vi "Reorder Analyzers Dialog.vi"(8 "error in":errorcluster, 11 "Analyzers.Process Cache":refnum<class "Controller Array.lvclass">) -> (0 "error out":errorcluster, 3 "Reordered Analyzers.Process Cache":refnum<class "Controller Array.lvclass">)   [LabVIEW 2020, in "RxnRover.lvlib"]
uses:
  RxnRover.lvlib
  Plugin Servers/Controller Array/Controller Array.lvclass
  Plugin Servers/Controller/Generic Plugin.lvclass/Generic Plugin.ctl
  Plugin Servers/Controller Array/Searchable Properties.ctl
  Plugin Servers/Controller/Generic Plugin.lvclass
panel:
  in  "Analyzer List":i32(listbox)
  out "Current Analyzer":string
  in  "Done":bool
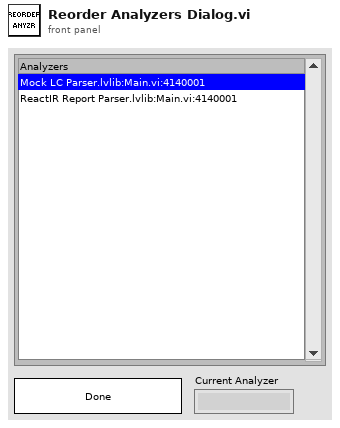
[diagram p1: front panel]
types:
  T1 = typedef "RxnRover.lvlib/Controller Array.lvclass/Searchable Properties.ctl" = enum16{"Name", "Controller Type"}
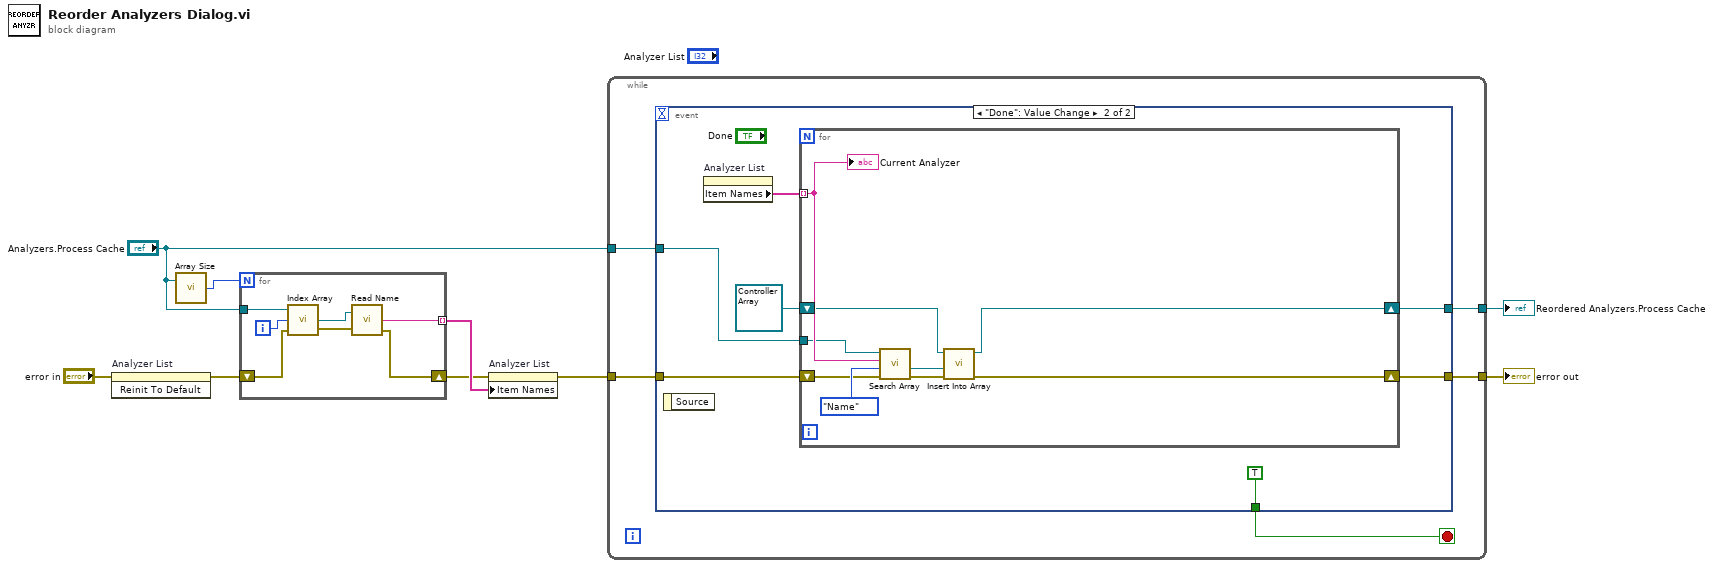
[diagram p0: block diagram]
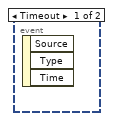
[diagram p2: hidden frame]
diagram:
  n1 = invoke on="Analyzer List" class="LstBox (strict)" method="Reinit To Default"(error in="error in") -> (error out=w7:errorcluster)  [unwired: 2 in, 2 out]
  n2 = call "Array Size.vi"("Controller Array in"="Analyzers.Process Cache") -> ("size(s)"=w9:i32)  [unwired: 1 in, 2 out]
  n3 = for {
    N: w9 -> [_]
    tunnel: "Analyzers.Process Cache" -> [w16]
    shift-right: [w12] -> w5
    shift-left: w7 -> [w11]
    tunnel: [w10] -> w6 mode=indexing
    i -> [w15]
    n4 = call "Index Array.vi"("error in (no error)"=w11, "index"=w15, "Controller Array in"=w16) -> ("error out"=w13:errorcluster, "element"=w14:refnum<class "Generic Plugin.lvclass">)  [unwired: 1 out]
    n5 = call "Read Name.vi"("controller in"=w14, "error in (no error)"=w13) -> ("Name"=w10:string, "error out"=w12:errorcluster)  [unwired: 1 out]
  }
  n6 = property on="Analyzer List" class="LstBox (strict)"(error in=w5, "Item Names"=w6) -> (error out=w4:errorcluster)  [unwired: 1 in, 1 out]
  n7 = while {
    tunnel: w4 -> [w19]
    tunnel: "Analyzers.Process Cache" -> [w20]
    tunnel: [w18] -> w2
    tunnel: [w17] -> w1
    stop <- w21 stop-if-true
    n8 = event shown="[1] \"Done\": Value Change" {
      selector: _ -> [_ _]
      dyn-events: _ -> [_ _]
      timeout: _ -> [_ _]
      tunnel: [_ TRUE] -> w21
      tunnel: w20 -> [_ w26]
      tunnel: w19 -> [_ w24]
      tunnel: [_ w23] -> w18
      tunnel: [_ w22] -> w17
      event Timeout {
        n9 = event-data() -> ()  [unwired: 1 in, 3 out]
      }
      event "Done": Value Change {
        n10 = event-data() -> ()  [unwired: 1 in, 1 out]
        n11 = property on="Analyzer List" class="LstBox (strict)"() -> ("Item Names"=w27:string[])  [unwired: 2 in, 2 out]
        n12 = for {
          tunnel: w27 -> [w37] mode=indexing
          tunnel: w26 -> [w36]
          shift-right: [w34] -> w22
          shift-left: w24 -> [w30]
          shift-right: [w32] -> w23
          shift-left: refnum<class "Controller Array.lvclass"> refnum ("Analyzers.Process Cache") -> [w33]
          n13 = call "Search Array.vi"("error in (no error)"=w30, "Searchable Property (Name)"=Searchable_Properties."Name", "Search Value"=w37, "Controller Array in"=w36) -> ("error out"=w29:errorcluster, "Controller found"=w35:refnum<class "Generic Plugin.lvclass">)  [unwired: 2 out]
          n14 = call "Insert Into Array.vi"("error in (no error)"=w29, "new element"=w35, "Controller Array in"=w33) -> ("error out"=w34:errorcluster, "Controller Array out"=w32:refnum<class "Controller Array.lvclass">)  [unwired: 2 in, 1 out]
          "Current Analyzer" <- w37
        }
      }
    }
  }
  "Reordered Analyzers.Process Cache" <- w2
  "error out" <- w1
